vi "Current Loop - NI 9505 (FPGA).vi"() -> ()   [LabVIEW 2013]
doc: "This VI shows an example of how to implement a current loop for use with the NI 9505. The VI consists of a closed loop PI system with PWM generation and error monitoring. The desired load current can be set and the loop will monitor the actual current and adjust the PWM duty cycle until the desired current is reached."
uses:
  <vilib>/LabVIEW Targets/FPGA/cRIO/cRIO-9505/controls.llb/_nicrio_cRIO-9505_DriveStatus.ctl
  <vilib>/Platform/TimedLoop/XDataNode/timing_clust.ctl
  <vilib>/Platform/TimedLoop/XDataNode/nitl_modes.ctl
  <vilib>/Platform/TimedLoop/XDataNode/wakeup.ctl
  <vilib>/LabVIEW Targets/FPGA/cRIO/cRIO-9505/controls.llb/_nicrio_cRIO-9505_DriveDirection.ctl
  <vilib>/rvi/Emulation/niFpgaSctlEmulationGetInTimedLoop.vi
  <vilib>/rvi/Emulation/niFpgaEmulationReportErrorSimple.vi
  <vilib>/rvi/Emulation/niFpgaGetClockAttributes.vi
  <vilib>/rvi/Emulation/niFpgaCriticalErrorInLSC.vi
  <vilib>/rvi/Emulation/niFpgaProcessEmulError.vi
  <vilib>/rvi/eio/common/nirviEmuTemplateMethod_errors.vi
  <vilib>/rvi/eio/common/nirviEmuTemplatePropertyGet_noerrors.vi
  Instance           1 37Saved   Current Loop - NI 9505 (FPGA) .vi
  <vilib>/Platform/TimedLoop/XDataNode/XDataNode.xnode
  <vilib>/eio/EIONode/EIONode.xnode
  <vilib>/eio/EIOMethodNode/EIOMethodNode.xnode
  <vilib>/eio/EIOPropertyNode/EIOPropertyNode.xnode
  <vilib>/addons/control/pid/fpga.llb/XNode/niFpgaPID.xnode
  <vilib>/rvi/FXPMathLib/FxpMul/XNode/nifxpmath_Multiplier.xnode
  <vilib>/Platform/TimedLoop/XDataNode/XDNodeRunTimeDep.lvlib
  <vilib>/rvi/eio/common/nirviEmuTemplatePropertyGet_errors.vi
  <vilib>/rvi/eio/common/nirviEmuTemplatePropertySet_errors.vi
  <vilib>/rvi/eio/common/nirviEmuTemplatePropertySet_noerrors.vi
  <vilib>/rvi/FXPMathLib/sim/FxpSim.dll
panel:
  in  "PID gains":T1={"proportional gain (Kc)"=1.0, "integral gain (Kc*Ts/Ti)"=1.66796875, "derivative gain (Kc*Td/Ts)"=0.0}
  out "output 2":i16
  out "output":i16
  out "x*y":fxp<+/-,28,13>
  out "PWM Duty Cycle":i16
  out "Measured Force (N)":fxp<+,39,10>
  in  "ForceSensorGain":fxp<+,21,7>=52.97296142578125 format="%#_10g"
  in  "L12 Gain (mA/N)":fxp<+,21,2>=1.0
  in  "L12 Offset (mA)":fxp<+,21,5>=1.0
  in  "Command Force (N)":fxp<+,16,6>
  in  "Disable\nDrive":bool
  in  "Enable\nDrive":bool
  out "Temp Fault":bool
  out "Drive Status":T2=enum."Disabled"
  out "Drive Fault":bool
  out "Vsup Present":bool
  in  "Current Loop\nRate (usec)":u32=50
  in  "Current Limit":i16 caption="Setpoint" min=0 max=2047
  in  "Current PI gains - (x 2^8)":T3={"Proportional Gain"=20, "Integral Gain"=10, "Derivative Gain"=0}
  in  "Current Setpoint":i16 caption="Setpoint"
  in  "Trig AI":bool
  in  "Current Feedback\nCounts":i16
  # "VI Execution\nThis VI should be run using \"Current Loop - NI 9505 (RT).vi\"."
  # "These parameters control the response\nof the current loop. The setpoint is the\ncommanded current and the limit is the\nmaximum current command allowed."
  # "These status controls/indicators are\nused to enable/disable the drive and\nread fault information."
  # "These three controls/indicators are\nused by the individual loops and should\nnot be changed."
  # "Drive Status"
  # "Current Loop Parameters"
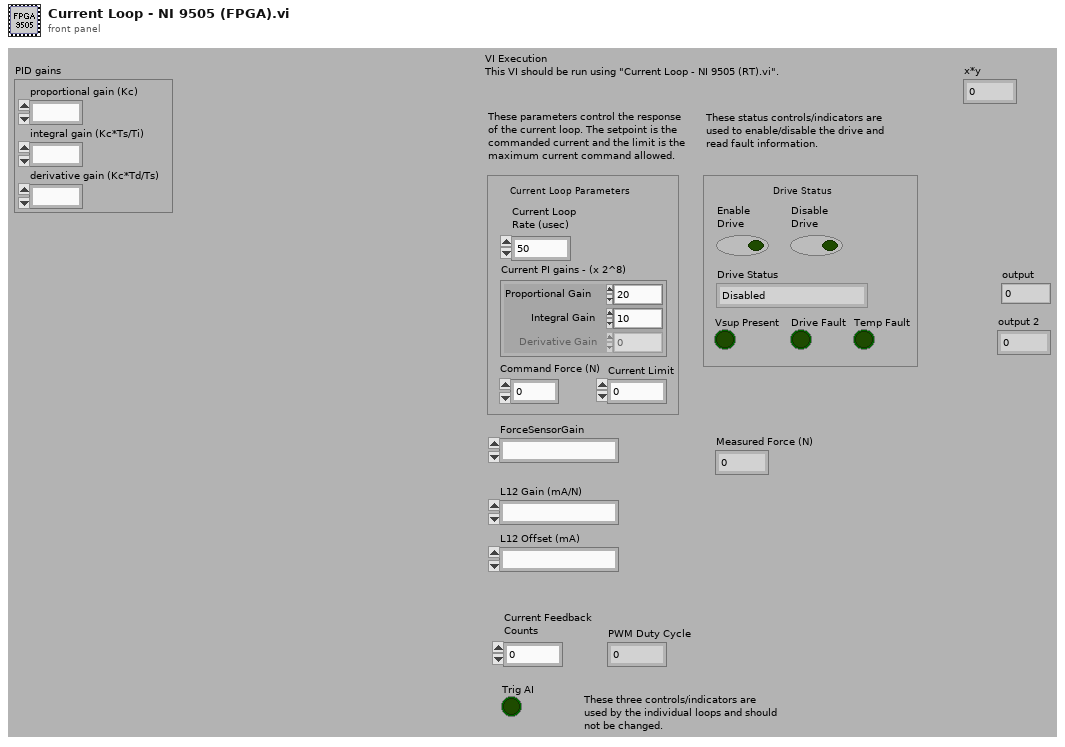
[diagram p1: front panel]
types:
  T1 = cluster{"proportional gain (Kc)":fxp<+/-,16,8>, "integral gain (Kc*Ts/Ti)":fxp<+/-,16,8>, "derivative gain (Kc*Td/Ts)":fxp<+/-,16,8>}
  T2 = typedef "_nicrio_cRIO-9505_DriveStatus.ctl" = enum8{"Enabled", "Disabled", "Disabled by Drive Fault", "Disabled by Temp. Fault", "Disabled by E-Stop", "Unknown"}
  T3 = cluster{"Proportional Gain":i16, "Integral Gain":i16, "Derivative Gain":i16}
  T4 = typedef "XDNodeRunTimeDep.lvlib/timing_clust.ctl" = cluster{"Expected End [f-1]":u64, "Actual End [f-1]":u64, "Finished Late? [f-1]":bool, "Expected End [i-1]":u64, "Actual End [i-1]":u64, "Finished Late? [i-1]":bool, "Expected Start [i]":u64, "Actual Start [i]":u64, "Expected Start [f]":u64, "Actual Start [f]":u64, "Source Name":string, "Structure Name":string, "Period":i64, "Deadline":i64, "Offset":i64, "Start":i64, "Priority":i32, "Timeout":i32, "Mode":T5, "Wakeup Reason":T6, "Error":errorcluster, "Source Type":string, "Secondary Source Type":string, "Global End Time":u64, "Global Start Time":u64, "Frame Duration":u64, "Iteration Duration":u64, "Assigned CPU":i32, "I/O Scan Engine Mode":u32}
  T5 = typedef "XDNodeRunTimeDep.lvlib/nitl_modes.ctl" = enum32{"No Change", "Process missed periods, maintain original phase", "Discard missed periods, maintain original phase", "Process missed periods, ignore original phase", "Discard missed periods, ignore original phase"}
  T6 = typedef "XDNodeRunTimeDep.lvlib/wakeup.ctl" = enum32{"Normal", "Aborted", "Asynchronous wakeup", "Timing source error", "Timed loop error", "Timeout"}
  T7 = typedef "_nicrio_cRIO-9505_DriveDirection.ctl" = enum8{"Clockwise", "Counterclockwise"}
  T8 = cluster{"proportional gain (Kc)":i16, "integral gain (Kc*Ts/Ti)":i16, "derivative gain (Kc*Td/Ts)":i16}
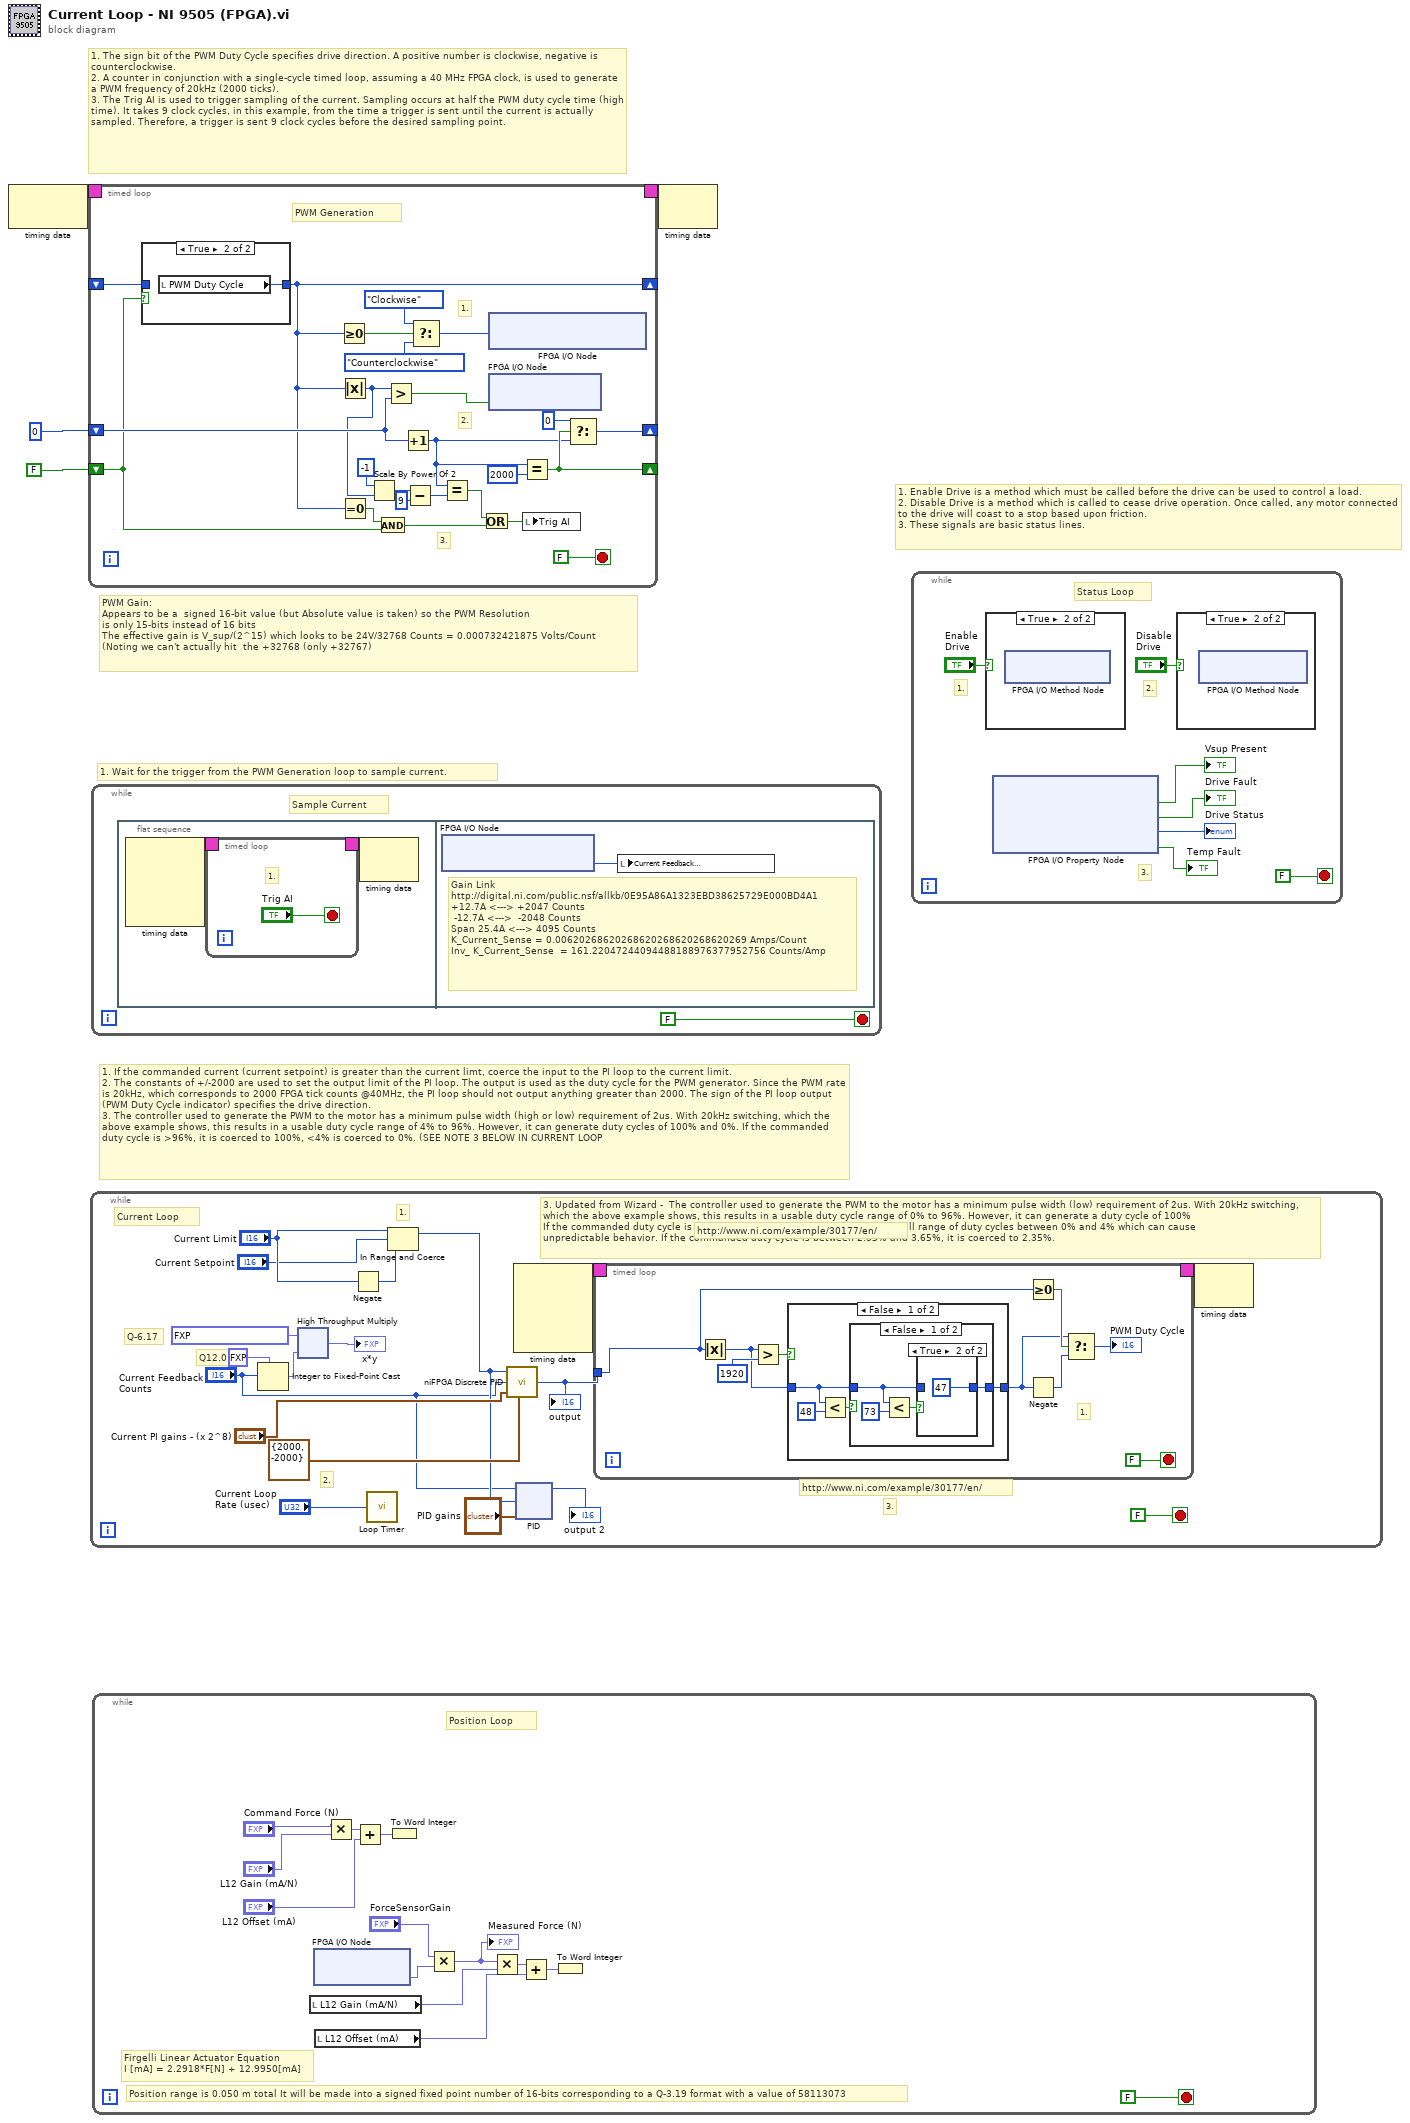
[diagram p0: block diagram]
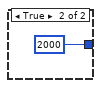
[diagram p7: hidden frame]
diagram:
  # "PWM Gain:\nAppears to be a  signed 16-bit value (but Absolute value is taken) so the PWM Resolution\nis only 15-bits instead of 16 bits\nThe effective gain is V_sup/(2^15) which looks to be 24V/32768 Counts = 0.000732421875 Volts/Count\n(Noting we can't actually hit  the +32768 (only +32767)"
  # "1. Enable Drive is a method which must be called before the drive can be used to control a load.\n2. Disable Drive is a method which is called to cease drive operation. Once called, any motor connected to the drive will coast to a stop based upon friction.\n3. These signals are basic status lines."
  # "1. Wait for the trigger from the PWM Generation loop to sample current."
  # "1. The sign bit of the PWM Duty Cycle specifies drive direction. A positive number is clockwise, negative is counterclockwise.\n2. A counter in conjunction with a single-cycle timed loop, assuming a 40 MHz FPGA clock, is used to generate a PWM frequency of 20kHz (2000 ticks).\n3. The Trig AI is used to trigger sampling of the current. Sampling occurs at half the PWM duty cycle time (high time). It takes 9 clock cycles, in this example, from the time a trigger is sent until the current is actually sampled. Therefore, a trigger is sent 9 clock cycles before the desired sampling point."
  # "1. If the commanded current (current setpoint) is greater than the current limt, coerce the input to the PI loop to the current limit.\n2. The constants of +/-2000 are used to set the output limit of the PI loop. The output is used as the duty cycle for the PWM generator. Since the PWM rate is 20kHz, which corresponds to 2000 FPGA tick counts @40MHz, the PI loop should not output anything greater than 2000. The sign of the PI loop output (PWM Duty Cycle indicator) specifies the drive direction.\n3. The controller used to generate the PWM to the motor has a minimum pulse width (high or low) requirement of 2us. With 20kHz switching, which the above example shows, this results in a usable duty cycle range of 4% to 96%. However, it can generate duty cycles of 100% and 0%. If the commanded duty cycle is >96%, it is coerced to 100%, <4% is coerced to 0%. (SEE NOTE 3 BELOW IN CURRENT LOOP"
  n1 = node-c288() -> (w4:T4)  [unwired: 1 out]
  n2 = timed-loop {
    timing: w4 -> [_]
    timing-out: [_] -> w3
    shift-right: [w25] -> _
    shift-left: i16 0 -> [w28]
    shift-right: [w24] -> _
    shift-left: FALSE -> [w21]
    shift-right: [w5] -> _
    shift-left: _ -> [w23]
    stop <- FALSE stop-if-true
    # "3."
    # "2."
    # "1."
    # "PWM Generation"
    n3 = case shown="True" w21 {
      tunnel: [w29 w30] -> w5
      tunnel: w23 -> [w29 _]
      frame False {
      }
      frame True {
        n4 = local read "PWM Duty Cycle"() -> (w30:i16)
      }
    }
    n5 = Greater Or Equal To 0?(x=w5) -> (x >= 0?=w17:bool)
    n6 = Absolute Value(x=w5) -> (abs(x)=w7:i16)
    n7 = Equal To 0?(x=w5) -> (x = 0?=w22:bool)
    n8 = Scale By Power Of 2(n=i8 -1, x=w7) -> (x*2^n=w10:i16)
    n9 = And(x=w22, y=w21) -> (x .and. y?=w18:bool)
    n10 = Greater?(x=w7, y=w28) -> (0:w14:bool)
    n11 = Increment(x=w28) -> (x+1=w20:i16)
    n12 = Subtract(x=w10, y=i8 9) -> (x-y=w9:i16)
    n13 = Select(t=_nicrio_cRIO-9505_DriveDirection."Clockwise" ("Drive Direction"), s=w17, f=_nicrio_cRIO-9505_DriveDirection."Counterclockwise" ("Drive Direction")) -> (s? t:f=w13:T7)
    n14 = Equal?(x=w20, y=w9) -> (x = y?=w19:bool)
    n15 = Or(x=w19, y=w18) -> (x .or. y?=w12:bool)
    n16 = xnode "FPGA I/O Node"("Mod2/Drive Direction"=w13) -> ()  [unwired: 1 in, 1 out]
    n17 = xnode "FPGA I/O Node"("Mod2/Motor"=w14) -> ()  [unwired: 1 in, 1 out]
    n18 = Equal?(x=w20, y=i16 2000) -> (x = y?=w24:bool)
    n19 = local write "Trig AI"(w12) -> ()
    n20 = Select(t=i16 0, s=w24, f=w20) -> (s? t:f=w25:i16)
  }
  n21 = while {
    stop <- FALSE stop-if-true
    # "Q12.0"
    # "Q-6.17"
    # "http://www.ni.com/example/30177/en/"
    # "3. Updated from Wizard -  The controller used to generate the PWM to the motor has a minimum pulse width (low) requirement of 2us. With 20kHz switching, which the above example shows, this results in a usable duty cycle range of 0% to 96%. However, it can generate a duty cycle of 100%\nIf the commanded duty cycle is >96%, it is coerced to 100%. There is a small range of duty cycles between 0% and 4% which can cause\nunpredictable behavior. If the commanded duty cycle is between 2.35% and 3.65%, it is coerced to 2.35%."
    # "http://www.ni.com/example/30177/en/"
    # "3."
    # "2."
    # "1."
    # "Current Loop"
    n22 = Integer to Fixed-Point Cast(fixed-point type=fxp<+/-,12,12> 0.0, integer="Current Feedback\nCounts") -> (fixed-point=w39:fxp<+/-,12,12>)
    n23 = xnode ("High Throughput Multiply")("x"=fxp<+/-,11,-6> 0.00620269775390625, "y"=w39) -> ("x*y"=→"x*y":fxp<+/-,23,6>)
    n24 = Negate(x="Current Limit") -> (-x=w48:i16)
    n25 = call "Loop Timer"("Count(uSec)"="Current Loop\nRate (usec)") -> ()  [unwired: 1 out]
    n26 = In Range and Coerce(upper limit="Current Limit", x="Current Setpoint", lower limit=w48) -> (coerced(x)=w36:i16)  [unwired: 1 out]
    n27 = call <vilib>:"niFPGA Discrete PID.vi"("setpoint"=w36, "process variable"="Current Feedback\nCounts", "PID gains (x 2^8)"="Current PI gains - (x 2^8)", "output range"=cluster{"output high":i16, "output low":i16} {"output high"=2000, "output low"=-2000}) -> ("output"=w41:i16)  [unwired: 1 in, 4 out]
    "output" <- w41
    n28 = node-c288() -> (w43:T4)  [unwired: 4 in]
    n29 = xnode "PID"("process variable"="Current Feedback\nCounts", "setpoint"=w36, "PID gains"="PID gains") -> ("output"=→"output 2":i16)  [unwired: 2 in]
    n30 = timed-loop {
      timing: w43 -> [_]
      timing-out: [_] -> w42
      tunnel: w41 -> [w79]
      stop <- FALSE stop-if-true
      # "1."
      n31 = Absolute Value(x=w79) -> (abs(x)=w82:i16)
      n32 = Greater?(x=w82, y=i16 1920 ("upper limit")) -> (0:w84:bool)
      n33 = case shown="False" w84 {
        tunnel: [w90 i16 2000 ("upper limit")] -> w83
        tunnel: w82 -> [w88 _]
        frame False {
          n34 = Less?(x=w88, y=i16 48 ("lower limit")) -> (x < y?=w89:bool)
          n35 = case shown="False" w89 {
            tunnel: [w92 w98] -> w90
            tunnel: w88 -> [w93 w98]
            frame False {
              n36 = Less?(x=w93, y=i16 73 ("lower limit")) -> (x < y?=w94:bool)
              n37 = case shown="True" w94 {
                tunnel: w93 -> [w96 _]
                tunnel: [w96 i16 47 ("lower limit")] -> w92
                frame False {
                }
                frame True {
                }
              }
            }
            frame True {
            }
          }
        }
        frame True {
        }
      }
      n38 = Greater Or Equal To 0?(x=w79) -> (x >= 0?=w87:bool)
      n39 = Negate(x=w83) -> (-x=w86:i16)
      n40 = Select(t=w83, s=w87, f=w86) -> (s? t:f=→"PWM Duty Cycle":i16)
    }
    n41 = node-c288(w42) -> ()  [unwired: 1 out]
  }
  n42 = while {
    stop <- FALSE stop-if-true
    # "Sample Current"
    n43 = flat-sequence {
      frame #0 {
        n44 = node-c288() -> (w106:T4)  [unwired: 4 out]
        n45 = timed-loop {
          timing: w106 -> [_]
          timing-out: [_] -> w105
          stop <- "Trig AI" stop-if-true
          # "1."
        }
        n46 = node-c288(w105) -> ()  [unwired: 1 out]
      }
      frame #1 {
        # "Gain Link\nhttp://digital.ni.com/public.nsf/allkb/0E95A86A1323EBD38625729E000BD4A1\n+12.7A <---> +2047 Counts\n -12.7A <--->  -2048 Counts\nSpan 25.4A <---> 4095 Counts\nK_Current_Sense = 0.00620268620268620268620268620269 Amps/Count\nInv_ K_Current_Sense  = 161.22047244094488188976377952756 Counts/Amp"
        n47 = xnode "FPGA I/O Node"() -> ("Mod2/Current Sense"=w112:i16)  [unwired: 1 in, 1 out]
        n48 = local write "Current Feedback\nCounts"(w112) -> ()
      }
    }
  }
  n49 = while {
    stop <- FALSE stop-if-true
    # "Position range is 0.050 m total It will be made into a signed fixed point number of 16-bits corresponding to a Q-3.19 format with a value of 58113073"
    # "Firgelli Linear Actuator Equation\nI [mA] = 2.2918*F[N] + 12.9950[mA]"
    # "Position Loop"
    n50 = local read "L12 Gain (mA/N)"() -> (w120:fxp<+,21,2>)
    n51 = xnode "FPGA I/O Node"() -> ("Mod1/AI0"=w117:fxp<+,18,3>)  [unwired: 1 in, 1 out]
    n52 = local read "L12 Offset (mA)"() -> (w121:fxp<+,21,5>)
    n53 = Multiply(x="Command Force (N)", y="L12 Gain (mA/N)") -> (x*y=w123:fxp<+,37,8>)
    n54 = Add(x=w123, y="L12 Offset (mA)") -> (x+y=w122:fxp<+,38,9>)
    n55 = To Word Integer(number=w122) -> ()  [unwired: 1 out]
    n56 = Multiply(x="ForceSensorGain", y=w117) -> (x*y=w114:fxp<+,39,10>)
    "Measured Force (N)" <- w114
    n57 = Multiply(x=w114, y=w120) -> (x*y=w118:fxp<+,60,12>)
    n58 = Add(x=w118, y=w121) -> (x+y=w119:fxp<+,61,13>)
    n59 = To Word Integer(number=w119) -> ()  [unwired: 1 out]
  }
  n60 = node-c288(w3) -> ()  [unwired: 1 out]
  n61 = while {
    stop <- FALSE stop-if-true
    # "3."
    # "2."
    # "1."
    # "Status Loop"
    n62 = case shown="True" "Enable\nDrive" {
      frame False {
      }
      frame True {
        n63 = xnode "FPGA I/O Method Node"() -> ()  [unwired: 1 in, 1 out]
      }
    }
    n64 = xnode "FPGA I/O Property Node"() -> ("Vsup Present"=→"Vsup Present":bool, "Drive Fault"=→"Drive Fault":bool, "Drive Status"=→"Drive Status":T2, "Over Temperature Fault"=→"Temp Fault":bool)  [unwired: 1 in, 1 out]
    n65 = case shown="True" "Disable\nDrive" {
      frame False {
      }
      frame True {
        n66 = xnode "FPGA I/O Method Node"() -> ()  [unwired: 1 in, 1 out]
      }
    }
  }
